vi "EnqueueWithAck.vi"(7 "Instance":i32, 8 "error in (no error)":errorcluster, 10 "Data":variant, 11 "Msg":string) -> (0 "error out":errorcluster, 2 "Response":variant)   [LabVIEW 2017, in "Communication.lvlib"]
uses:
  Communication.lvlib
  SubVIs/MsgData.ctl
  SubVIs/MsgAck.ctl
panel:
  in  "timeout in ms (-1)":i32=500
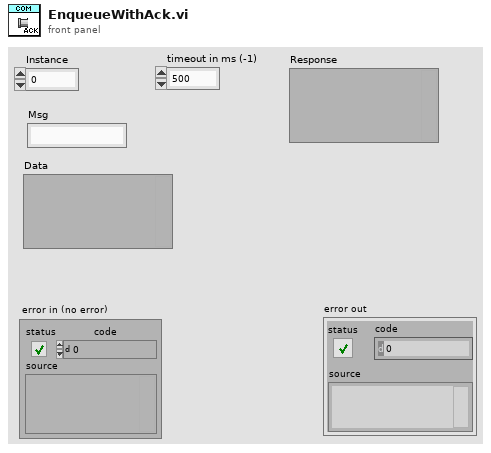
[diagram p1: front panel]
types:
  T1 = typedef "Communication.lvlib/MsgAck.ctl" = cluster{"Variant":variant, "error ":errorcluster}
  T2 = typedef "Communication.lvlib/MsgData.ctl" = cluster{"Msg":string, "Data":variant, "Ack":refnum<notifier>}
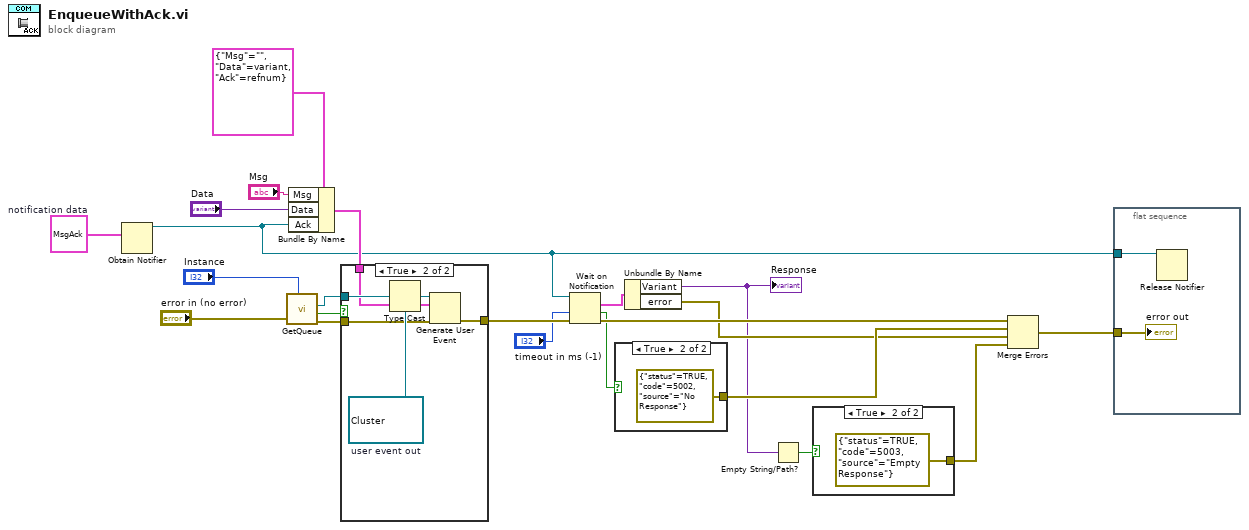
[diagram p0: block diagram]
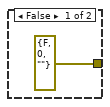
[diagram p2: hidden frame]
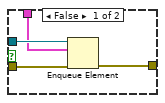
[diagram p3: hidden frame]
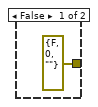
[diagram p4: hidden frame]
diagram:
  w14 = T1 {"Variant"=variant, "error "={"status"=FALSE, "code"=0, "source"=""}}  # notification data
  n1 = Obtain Notifier(notification data type=w14) -> (notifier out=w8:refnum<notifier>)  [unwired: 3 in, 2 out]
  n2 = call "GetQueue.vi"("Instance"="Instance", "error in (no error)"="error in (no error)") -> ("error out"=w20:errorcluster, "Event?"=w4:bool, "queue out"=w19:refnum<queue>)  [unwired: 7 in]
  n3 = Bundle By Name(cluster=T2 {"Msg"="", "Data"=variant, "Ack"=refnum} ("element"), "Msg"="Msg", "Data"="Data", "Ack"=w8) -> (w17:T2)
  n4 = case shown="True" w4 {
    tunnel: w20 -> [w26 w27]
    tunnel: w19 -> [w25 w32]
    tunnel: w17 -> [w24 w28]
    tunnel: [w23 w30] -> w13
    frame False {
      n5 = Enqueue Element(queue=w25, element=w24, error in (no error)=w26) -> (error out=w23:errorcluster)  [unwired: 1 in, 2 out]
    }
    frame True {
      w31 = refnum<user-event> refnum  # user event out
      n6 = Type Cast(type=w31, x=w32) -> (*(type *) &x=w29:refnum<user-event>)
      n7 = Generate User Event(user event=w29, event data cluster=w28, error in=w27) -> (error out=w30:errorcluster)  [unwired: 1 in, 1 out]
    }
  }
  n8 = Wait on Notification(notifier=w8, timeout in ms (-1)="timeout in ms (-1)", error in (no error)=w13) -> (notification=w11:T1, timed out?=w9:bool, error out=w10:errorcluster)  [unwired: 1 in, 1 out]
  n9 = case shown="True" w9 {
    tunnel: [errorcluster {"status"=FALSE, "code"=0, "source"=""} ("error constant") errorcluster {"status"=TRUE, "code"=5002, "source"="No Response"} ("error constant")] -> w6
    frame False {
    }
    frame True {
    }
  }
  n10 = Unbundle By Name(w11) -> ("Variant"=w3:variant, "error"=w5:errorcluster)
  "Response" <- w3
  n11 = Empty String/Path?(string/path=w3) -> (empty?=w2:bool)
  n12 = case shown="True" w2 {
    tunnel: [errorcluster {"status"=FALSE, "code"=0, "source"=""} ("error constant") errorcluster {"status"=TRUE, "code"=5003, "source"="Empty Response"} ("error constant")] -> w1
    frame False {
    }
    frame True {
    }
  }
  n13 = Merge Errors(w10, w6, w5, w1) -> (w7:errorcluster)
  n14 = flat-sequence {
    tunnel: w8 -> [w38]
    tunnel: w7 -> [w37]
    frame #0 {
      n15 = Release Notifier(notifier=w38) -> ()  [unwired: 2 in, 3 out]
      "error out" <- w37
    }
  }
